vi "numbers in words.vi"() -> ()   [LabVIEW 2018]
panel:
  out "String":string
  in  "Numeric":dbl
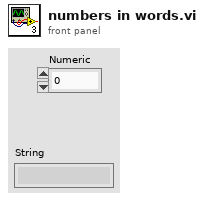
[diagram p1: front panel]
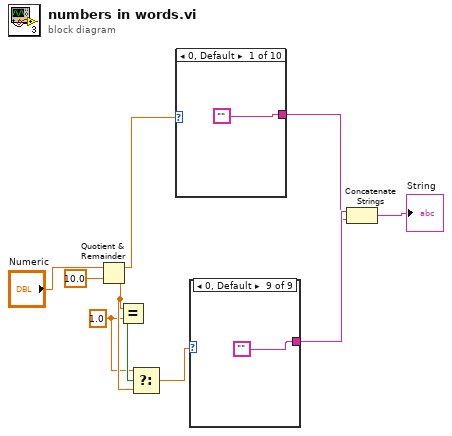
[diagram p0: block diagram]
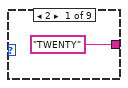
[diagram p2: hidden frame]
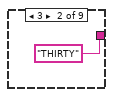
[diagram p3: hidden frame]
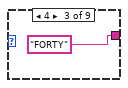
[diagram p4: hidden frame]
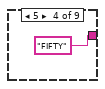
[diagram p5: hidden frame]
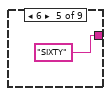
[diagram p6: hidden frame]
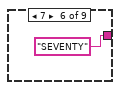
[diagram p7: hidden frame]
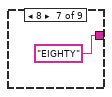
[diagram p8: hidden frame]
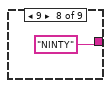
[diagram p9: hidden frame]
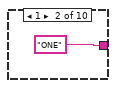
[diagram p10: hidden frame]
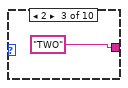
[diagram p11: hidden frame]
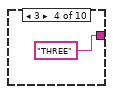
[diagram p12: hidden frame]
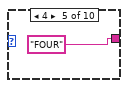
[diagram p13: hidden frame]
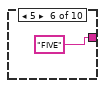
[diagram p14: hidden frame]
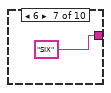
[diagram p15: hidden frame]
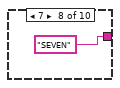
[diagram p16: hidden frame]
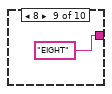
[diagram p17: hidden frame]
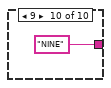
[diagram p18: hidden frame]
diagram:
  w3 = 1.0 ("y")
  n1 = Quotient & Remainder(x="Numeric", y=10.0) -> (x-y*floor(x/y)=w8:dbl, floor(x/y)=w5:dbl)
  n2 = Equal?(x=w5, y=w3) -> (x = y?=w6:bool)
  n3 = Select(t=w3, s=w6, f=w5) -> (s? t:f=w4:dbl)
  n4 = case shown="0, Default" w8 {
    tunnel: ["" "ONE" "TWO" "THREE" "FOUR" "FIVE" "SIX" "SEVEN" "EIGHT" "NINE"] -> w1
    frame 0, Default {
    }
    frame 1 {
    }
    frame 2 {
    }
    frame 3 {
    }
    frame 4 {
    }
    frame 5 {
    }
    frame 6 {
    }
    frame 7 {
    }
    frame 8 {
    }
    frame 9 {
    }
  }
  n5 = case shown="0, Default" w4 {
    tunnel: ["TWENTY" "THIRTY" "FORTY" "FIFTY" "SIXTY" "SEVENTY" "EIGHTY" "NINTY" ""] -> w2
    frame 2 {
    }
    frame 3 {
    }
    frame 4 {
    }
    frame 5 {
    }
    frame 6 {
    }
    frame 7 {
    }
    frame 8 {
    }
    frame 9 {
    }
    frame 0, Default {
    }
  }
  n6 = Concatenate Strings(w2, w1) -> (→"String":string)
